vi "StoreOutputMode.vi"(8 "error in (no error)":errorcluster, 9 "eOutputMode":u16(ring) items=["Function", "Arbitrary", "Sequence"], 11 "ClassIn":refnum<class "NISTFGenPluginsBase.lvclass">) -> (0 "error out":errorcluster, 3 "ClassOut":refnum<class "NISTFGenPluginsBase.lvclass">)   [LabVIEW 2014, in "FGenPlugins.lvlib" / "NISTFGenPluginsBase.lvclass"]
uses:
  NISTFGenPluginsBase.lvclass
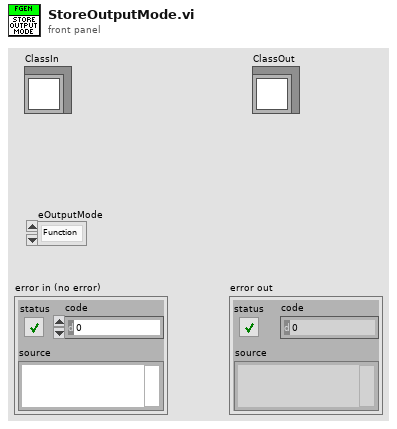
[diagram p1: front panel]
types:
  T1 = typedef "FGenPlugins.lvlib/NISTFGenPluginsBase.lvclass/ChannelParamElement.ctl" = cluster{"sName":string, "eOperateMode":u16, "bEnabled":bool, "eOutputMode":u16, "iIndex":i32, "iNameBufferSize":i32, "fGain":dbl}
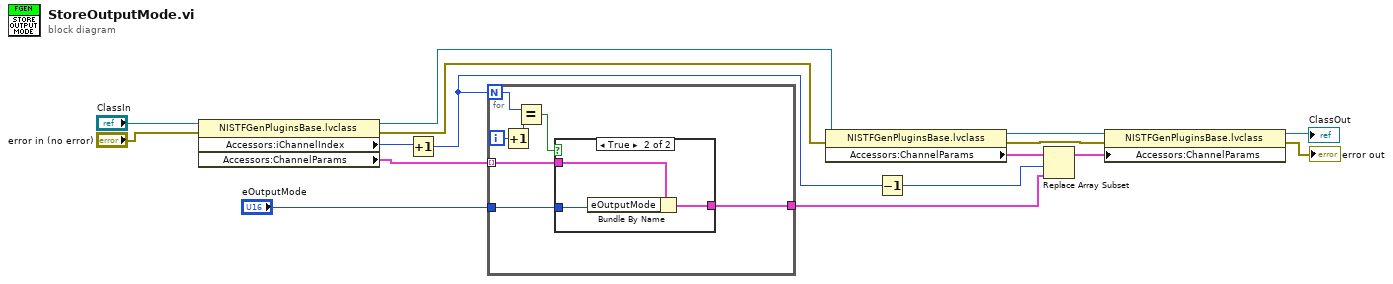
[diagram p0: block diagram]
diagram:
  n1 = property class="NISTFGenPluginsBase.lvclass"(reference="ClassIn", error in="error in (no error)") -> (reference out=w14:refnum<class "NISTFGenPluginsBase.lvclass">, error out=w7:errorcluster, "Accessors:iChannelIndex"=w3:i32, "Accessors:ChannelParams"=w15:T1[])
  n2 = Increment(x=w3) -> (x+1=w2:i32)
  n3 = for {
    N: w2 -> [w23]
    tunnel: w15 -> [w21] mode=indexing
    tunnel: "eOutputMode" -> [w20]
    tunnel: [w19] -> w12
    i -> [w18]
    n4 = Increment(x=w18) -> (x+1=w17:i32)
    n5 = Equal?(x=w23, y=w17) -> (x = y?=w22:bool)
    n6 = case shown="True" w22 {
      tunnel: w21 -> [w24 w27]
      tunnel: w20 -> [_ w26]
      tunnel: [w24 w25] -> w19
      frame False {
      }
      frame True {
        n7 = Bundle By Name(cluster=w27, "eOutputMode"=w26) -> (w25:T1)
      }
    }
  }
  n8 = property class="NISTFGenPluginsBase.lvclass"(reference=w14, error in=w7) -> (reference out=w11:refnum<class "NISTFGenPluginsBase.lvclass">, error out=w6:errorcluster, "Accessors:ChannelParams"=w13:T1[])
  n9 = Decrement(x=w2) -> (x-1=w1:i32)
  n10 = Replace Array Subset(array=w13, new element=w12, index=w1) -> (w10:T1[])
  n11 = property class="NISTFGenPluginsBase.lvclass"(reference=w11, error in=w6, "Accessors:ChannelParams"=w10) -> (reference out=→"ClassOut":refnum<class "NISTFGenPluginsBase.lvclass">, error out=→"error out":errorcluster)
